vi "HEWH Check Data Build String.vi"(8 "error in (no error)":errorcluster, 10 "Check Array":bool[](array[boolean]), 11 "Error Input":string) -> (0 "error out":errorcluster, 3 "Error Output":string)   [LabVIEW 2023]
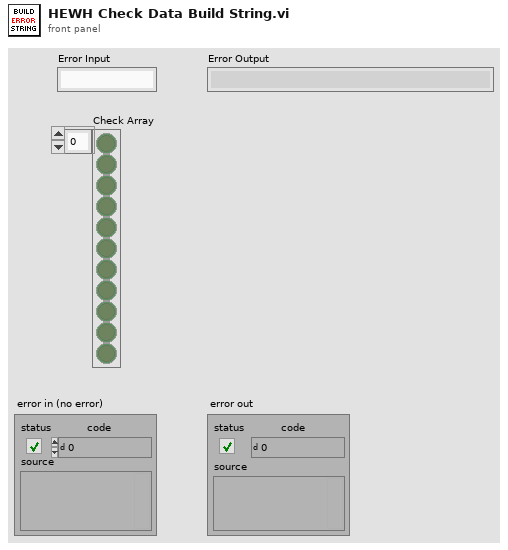
[diagram p1: front panel]
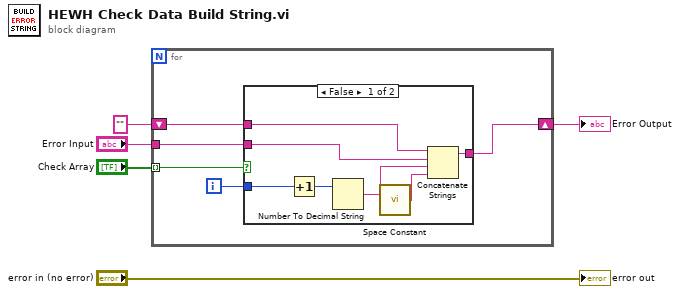
[diagram p0: block diagram]
diagram:
  n1 = for {
    tunnel: "Check Array" -> [w9] mode=indexing
    shift-right: [w8] -> w4
    shift-left: "" -> [w7]
    tunnel: "Error Input" -> [w6]
    i -> [w10]
    n2 = case shown="False" w9 {
      tunnel: w10 -> [w17 _]
      tunnel: [w14 w18] -> w8
      tunnel: w7 -> [w13 w18]
      tunnel: w6 -> [w11 _]
      frame False {
        n3 = Increment(x=w17) -> (x+1=w16:i32)
        n4 = Number To Decimal String(number=w16) -> (decimal integer string=w15:string)  [unwired: 1 in]
        n5 = call <vilib>:"Space Constant.vi"() -> ("String"=w12:string)
        n6 = Concatenate Strings(w13, w11, w15, w12) -> (w14:string)
      }
      frame True {
      }
    }
  }
  "Error Output" <- w4
  "error out" <- "error in (no error)"
